vi "Windows Message Queue Example.vi"() -> ()   [LabVIEW 2011]
doc: "This VI demonstrates the use of the Windows Message Queue,\nwhich allows for VIs to be sensitized to specified Windows\nMessages so that they can programmatically respond to the\nmessage.\n\n The call to Create Windows Message Queue configures this VI\nto receive mouse move, left button down and right button down\nmessages. The Wait for Windows Messages waits for the next\nmessage asynchronously. Upon its receipt, it sends all messages\ncurrently in the queue to the case structure that processes them.\n\nIf the Wait times out, we also remove all messages from the\nqueue. This is to prevent messages from building up in the\nqueue when they are not immediately handled. It ensures that\nall messages are processed as soon as possible. \nIt also ensures that if no further messages are received, we still\nprocess the ones currently in the queue after timing out on \nthe Wait.\n\nIf the user clicks in \"Click here to Exit,\" the while loop exits and\nthe Windows message queue is destroyed."
panel:
  out "Mouse Position":cluster{"X ":u16, "Y":u16}
  # "Bitmap picture"
  # "This VI demonstrates the use of the Windows Message Queue,\nwhich allows for VIs to be sensitized to specified Windows\nMessages so that they can programmatically respond to the\nmessage.\n\n The call to Create Windows Message Queue configures this VI\nto receive mouse move, left button down and right button down\nmessages.  The Wait for Windows Messages waits for the next\nmessage asynchronously.  Upon its receipt, it sends all messages\ncurrently in the queue to the case structure that processes them.\n\nIf the Wait times out, we also remove all messages from the\nqueue.  This is to prevent messages from building up in the\nqueue when they are not immediately handled.  It ensures that\nall messages are processed as soon as possible. \nIt also ensures that if no further messages are received, we still\nprocess the ones currently in the queue after timing out on \nthe Wait.\n\nIf the user clicks in \"Click here to Exit,\" the while loop exits and\nthe Windows message queue is destroyed."
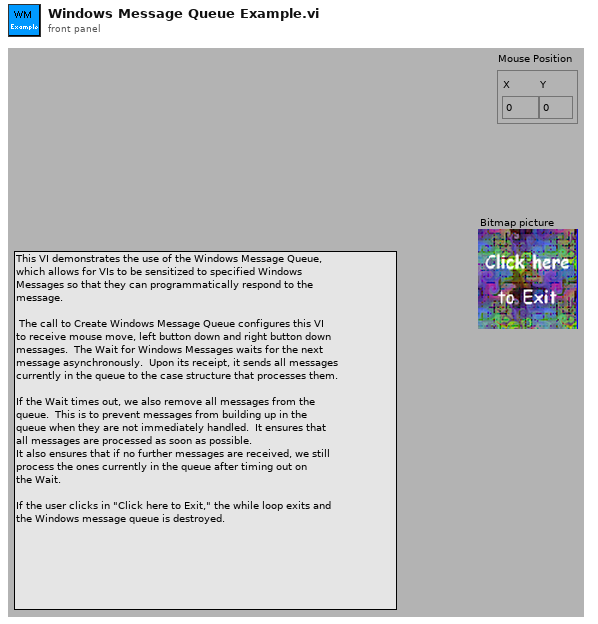
[diagram p1: front panel]
types:
  T1 = typedef "Win Msg Queue RefNum" = refnum<k1>
  T2 = cluster{"hWnd":u32, "Msg":u32, "wParam":u32, "lParam":i32, "time":u32, "point":cluster{"X":i32, "Y":i32}}
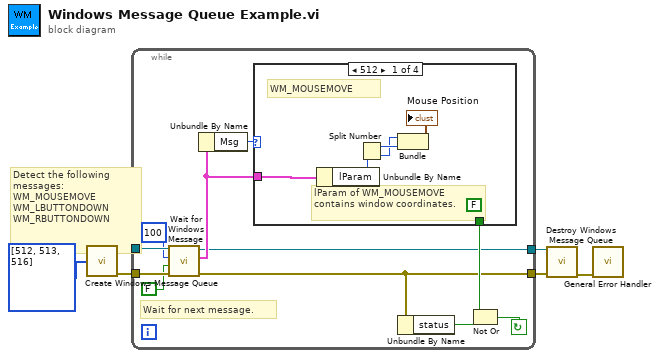
[diagram p0: block diagram]
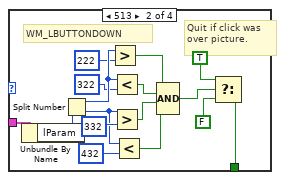
[diagram p2: hidden frame]
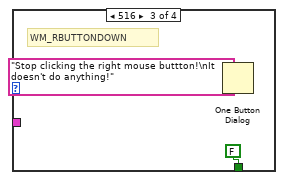
[diagram p3: hidden frame]
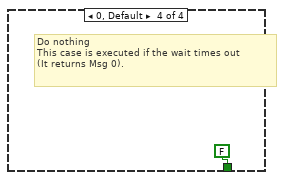
[diagram p4: hidden frame]
diagram:
  # "Detect the following\nmessages:\nWM_MOUSEMOVE\nWM_LBUTTONDOWN\nWM_RBUTTONDOWN"
  n1 = call "Create Windows Message Queue.vi"("Messeges (none)"=u32[] [512, 513, 516]) -> ("error out"=w4:errorcluster, "win msg queue"=w5:T1)  [unwired: 2 in]
  n2 = while {
    tunnel: [w8] -> w1
    tunnel: [w10] -> w2
    tunnel: w4 -> [w16]
    tunnel: w5 -> [w17]
    stop <- w15 continue-if-true
    # "Wait for next message."
    n3 = call "Wait for Windows Message.vi"("win msg queue"=w17, "ms timeout (-1)"=100, "ignore previous (F)"=FALSE ("ignore previous (T)"), "error in (no error)"=w16) -> ("win msg queue out"=w8:T1, "Message"=w9:T2, "error out"=w10:errorcluster)  [unwired: 3 out]
    n4 = Unbundle By Name(w9) -> ("Msg"=w7:u32)
    n5 = case shown="512" w7 {
      tunnel: [FALSE w26 FALSE FALSE] -> w12
      tunnel: w9 -> [w19 w25 _ _]
      frame 512 {
        # "WM_MOUSEMOVE"
        # "lParam of WM_MOUSEMOVE\ncontains window coordinates."
        n6 = Unbundle By Name(w19) -> ("lParam"=w18:i32)
        n7 = Split Number(x=w18) -> (hi(x)=w22:u16, lo(x)=w21:u16)
        n8 = Bundle(w21, w22) -> (→"Mouse Position":cluster{u16, u16})  [unwired: 1 in]
      }
      frame 513 {
        # "Quit if click was\nover picture."
        # "WM_LBUTTONDOWN"
        n9 = Unbundle By Name(w25) -> ("lParam"=w24:i32)
        n10 = Split Number(x=w24) -> (hi(x)=w36:u16, lo(x)=w38:u16)
        n11 = Greater?(x=w36, y=u16 222) -> (0:w33:bool)
        n12 = Less?(x=w36, y=u16 322) -> (x < y?=w32:bool)
        n13 = Greater?(x=w38, y=u16 332) -> (0:w31:bool)
        n14 = Less?(x=w38, y=u16 432) -> (x < y?=w30:bool)
        n15 = Compound Arithmetic op=AND(w33, w32, w31, w30) -> (w29:bool)
        n16 = Select(t=TRUE, s=w29, f=FALSE) -> (s? t:f=w26:bool)
      }
      frame 516 {
        # "WM_RBUTTONDOWN"
        n17 = One Button Dialog(message="Stop clicking the right mouse buttton!\nIt doesn't do anything!") -> ()  [unwired: 1 in, 1 out]
      }
      frame 0, Default {
        # "Do nothing\nThis case is executed if the wait times out\n(It returns Msg 0)."
      }
    }
    n18 = Unbundle By Name(w10) -> ("status"=w11:bool)
    n19 = Not Or(1:w11, 2:w12) -> (0:w15:bool)
  }
  n20 = call "Destroy Windows Message Queue.vi"("error in (no error)"=w2, "win msg queue"=w1) -> ("error out"=w3:errorcluster)
  n21 = call <vilib>:"General Error Handler.vi"("error in (no error)"=w3) -> ()  [unwired: 10 in, 5 out]
